vi "Write Boot code Version.vi"(8 "error in (no error)":errorcluster, 10 "Boot code Version":string, 11 "Lutron QS Object in":refnum<class "Lutron QS Object.lvclass">) -> (0 "error out":errorcluster, 3 "Lutron QS Object out":refnum<class "Lutron QS Object.lvclass">)   [LabVIEW 2016, in "Lutron QS Control Protocol.lvlib" / "Lutron QS Object.lvclass"]
uses:
  Lutron QS Object.lvclass
  Lutron QS Object.lvclass/Lutron QS Object.ctl
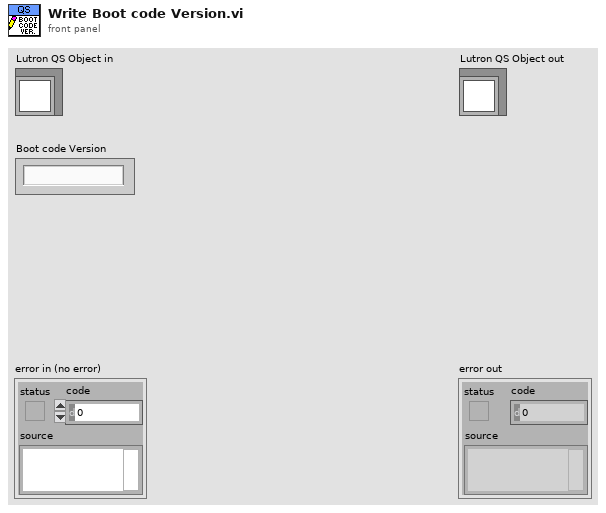
[diagram p1: front panel]
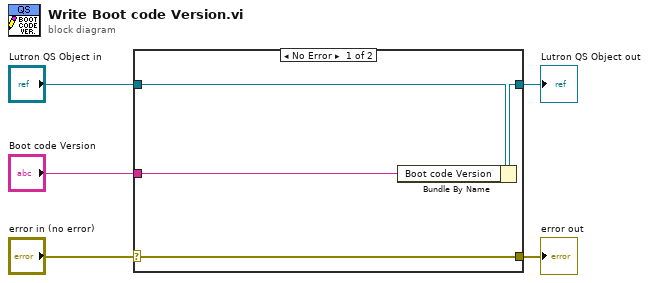
[diagram p0: block diagram]
diagram:
  n1 = case shown="No Error" "error in (no error)" {
    selector: "error in (no error)" -> [w9 w10]
    tunnel: [w9 w10] -> w4
    tunnel: [w7 w11] -> w2
    tunnel: "Lutron QS Object in" -> [w8 w11]
    tunnel: "Boot code Version" -> [w6 _]
    frame No Error {
      n2 = Bundle By Name(cluster=w8, "Boot code Version"=w6) -> (w7:refnum<class "Lutron QS Object.lvclass">)
    }
    frame Error {
    }
  }
  "error out" <- w4
  "Lutron QS Object out" <- w2
